vi "Servo_serial_mac_1readwrite.vi"() -> ()   [LabVIEW 2017]
uses:
  <vilib>/Instr/_visa.llb/VISA Configure Serial Port (Instr).vi
panel:
  in  "Pulse Width Input (600-2400)":dbl
  out "Servo Digital Signal":cluster{i32, dbl, dbl[]}(graph)
  out "Position Input":cluster{i32, dbl, dbl[]}(graph)
  out "Digitial Signal":dbl
  in  "Delay":dbl
  in  "Buad Rate":i32(ring) items=["2400"=2400, "4800"=4800, "9600"=9600, "14400"=14400, "19200"=19200, "28800"=28800, "38400"=38400, "57600"=57600, "115200"=115200]
  out "Bytes at port":cluster{i32, dbl, dbl[]}(graph)
  out "Read buffer":string
  in  "Stop":bool
  out "Sent to Arduino":string
  in  "COM Port":refnum<visa-resource-name>
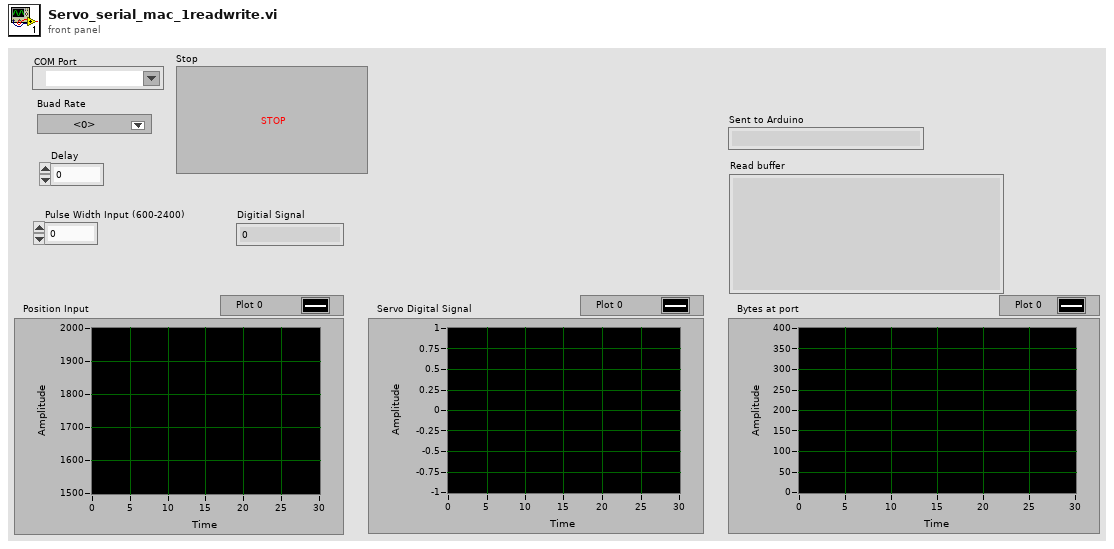
[diagram p1: front panel]
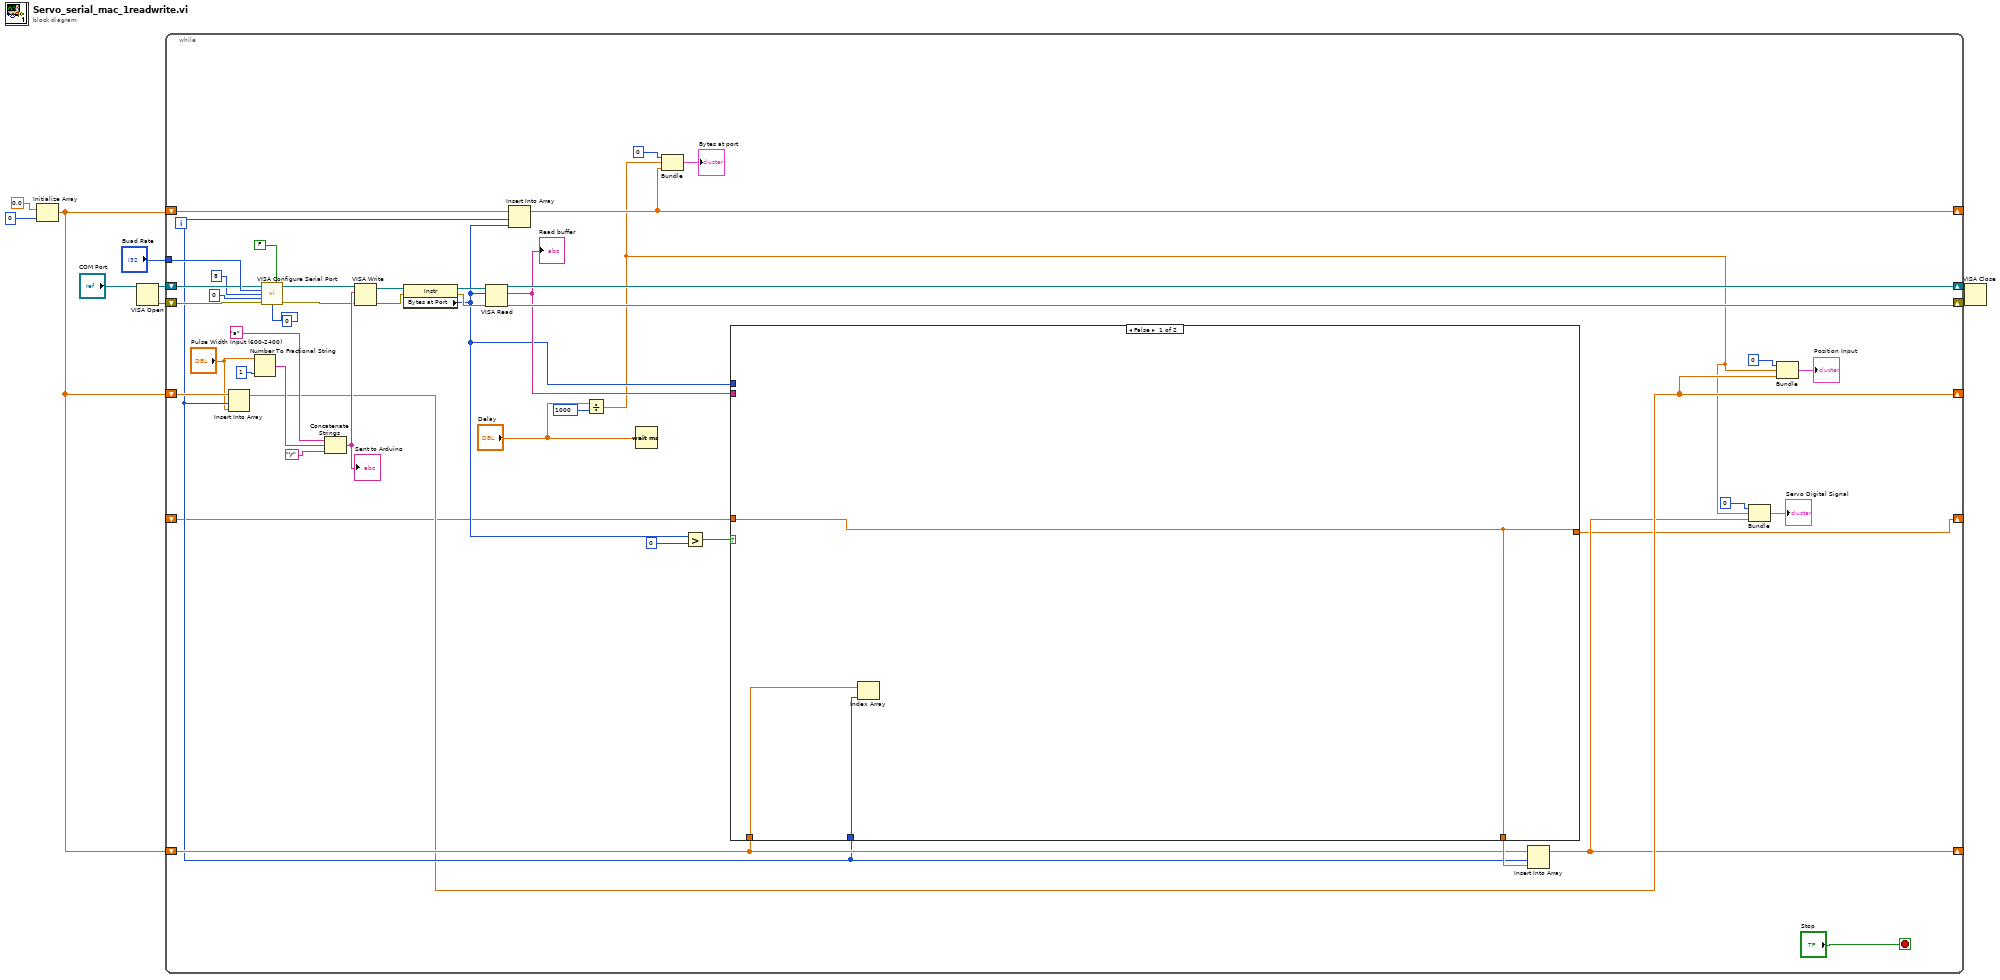
[diagram p0: block diagram]
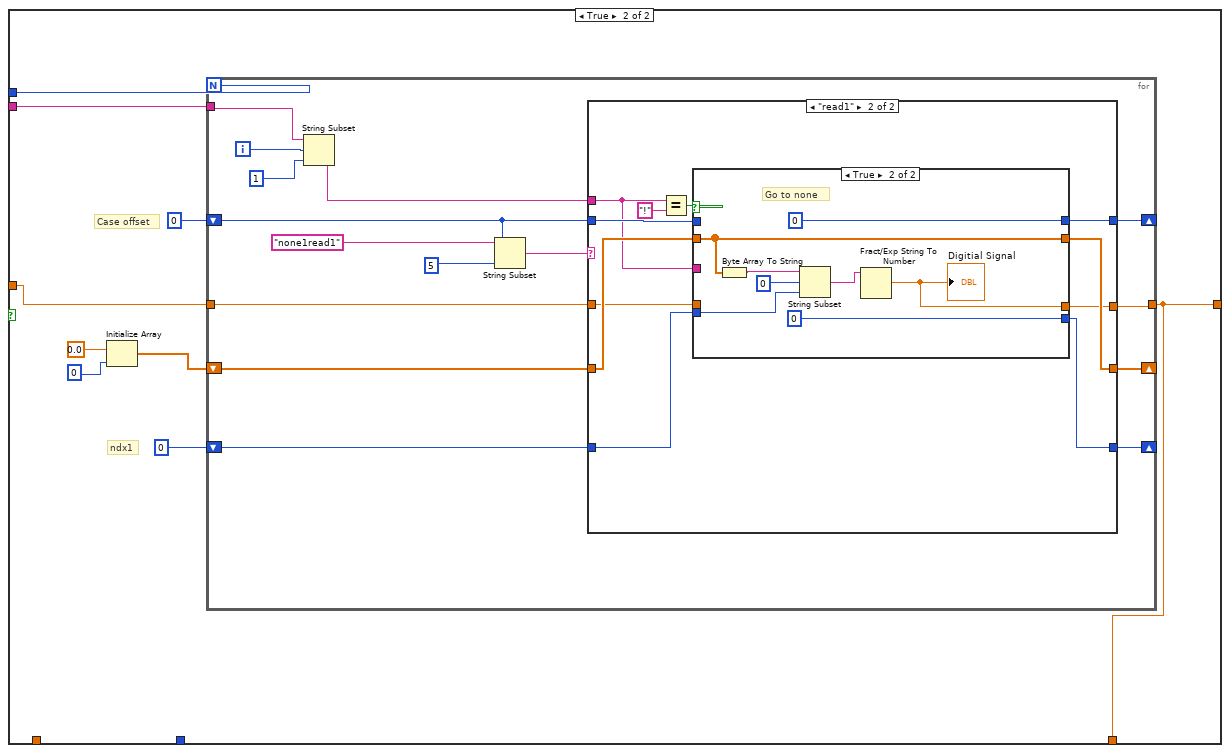
[diagram p2: hidden frame]
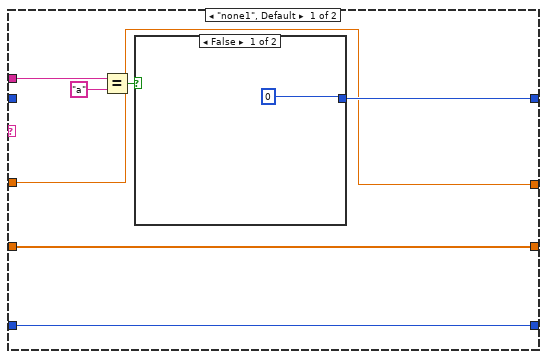
[diagram p3: hidden frame]
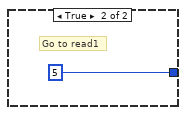
[diagram p4: hidden frame]
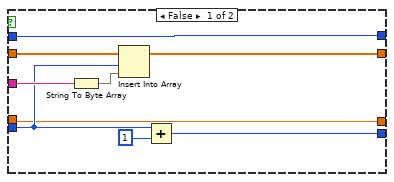
[diagram p5: hidden frame]
diagram:
  n1 = Initialize Array(0.0 ("element"), 0 ("dimension size")) -> (w1:dbl[])
  n2 = VISA Open(VISA resource name="COM Port") -> (VISA resource name=w8:refnum<visa-resource-name>, error out=w7:errorcluster)  [unwired: 4 in]
  n3 = while {
    tunnel: "Buad Rate" -> [w54]
    shift-right: [w50] -> w6
    shift-left: w8 -> [w53]
    shift-right: [w51] -> w5
    shift-left: w7 -> [w52]
    shift-right: [w48] -> _
    shift-left: w1 -> [w49]
    shift-right: [w19] -> _
    shift-left: w1 -> [w28]
    shift-right: [w18] -> _
    shift-left: w1 -> [w24]
    shift-right: [w14] -> _
    shift-left: _ -> [w15]
    i -> [w23]
    stop <- "Stop" stop-if-true
    n4 = Insert Into Array(array=w28, index=w23, new element="Pulse Width Input (600-2400)") -> (w19:dbl[])
    n5 = Number To Fractional String(number="Pulse Width Input (600-2400)", precision (6)=1) -> (F-format string=w44:string)  [unwired: 2 in]
    n6 = call-poly "VISA Configure Serial Port"("VISA resource name"=w53, "Enable Termination\nChar (T)"=FALSE ("Enable Termination\nChar (T)"), "baud rate (9600)"=w54, "data bits (8)"=8, "parity (0:none)"=0, "error in (no error)"=w52, "flow control (0:none)"=0) -> ("VISA resource name out"=w42:refnum<visa-resource-name>, "error out"=w45:errorcluster)  [unwired: 7 in]
    n7 = Concatenate Strings("a", w44, "\r") -> (w46:string)
    "Sent to Arduino" <- w46
    n8 = VISA Write(VISA resource name=w42, write buffer=w46, error in (no error)=w45) -> (VISA resource name out=w38:refnum<visa-resource-name>, error out=w41:errorcluster)  [unwired: 1 out]
    n9 = property class="Instr"(reference=w38, error in=w41) -> (reference out=w39:refnum<visa-resource-name>, error out=w40:errorcluster, "Bytes at Port"=w32:u32)
    n10 = VISA Read(VISA resource name=w39, byte count=w32, error in (no error)=w40) -> (VISA resource name out=w50:refnum<visa-resource-name>, read buffer=w34:string, error out=w51:errorcluster)  [unwired: 1 out]
    "Read buffer" <- w34
    n11 = Insert Into Array(array=w49, index=w23, new element=w32) -> (w48:dbl[])
    n12 = Divide(x="Delay", y=1000) -> (x/y=w17:dbl)
    n13 = Wait (ms)(milliseconds to wait="Delay") -> ()  [unwired: 1 out]
    n14 = Bundle(0, w17, w48) -> (→"Bytes at port":cluster{i32, dbl, dbl[]})  [unwired: 1 in]
    n15 = Greater?(x=w32, y=0) -> (0:w31:bool)
    n16 = case shown="False" w31 {
      tunnel: w32 -> [_ w60]
      tunnel: w34 -> [_ w66]
      tunnel: [w55 w58] -> w25
      tunnel: w23 -> [w56 _]
      tunnel: w24 -> [w57 _]
      tunnel: w15 -> [w55 w59]
      tunnel: [w55 w58] -> w14
      frame False {
        n17 = Index Array(array=w57, index=w56) -> ()  [unwired: 1 out]
      }
      frame True {
        # "ndx1"
        # "Case offset"
        n18 = Initialize Array(0.0 ("element"), 0 ("dimension size")) -> (w61:dbl[])
        n19 = for {
          N: w60 -> [_]
          tunnel: w66 -> [w80]
          shift-right: [w76] -> _
          shift-left: 0 -> [w70]
          shift-right: [w75] -> _
          shift-left: 0 -> [w74]
          shift-right: [w72] -> _
          shift-left: w61 -> [w73]
          tunnel: w59 -> [w67]
          tunnel: [w68] -> w58
          i -> [w69]
          n20 = String Subset(string=w80, offset (0)=w69, length (rest)=1 ("length (rest)")) -> (substring=w77:string)
          n21 = String Subset(string="none1read1", offset (0)=w70, length (rest)=5 ("length (rest)")) -> (substring=w71:string)
          n22 = case shown="\"read1\"" w71 {
            tunnel: w77 -> [w88 w91]
            tunnel: [w85 w98] -> w76
            tunnel: [w84 w94] -> w75
            tunnel: w74 -> [w84 w95]
            tunnel: w73 -> [w82 w96]
            tunnel: [w82 w99] -> w72
            tunnel: w70 -> [_ w97]
            tunnel: [w83 w93] -> w68
            tunnel: w67 -> [w83 w92]
            frame "none1", Default {
              n23 = Equal?(x=w88, y="a") -> (x = y?=w86:bool)
              n24 = case shown="False" w86 {
                tunnel: [0 5] -> w85
                frame False {
                }
                frame True {
                  # "Go to read1"
                }
              }
            }
            frame "read1" {
              n25 = Equal?(x=w91, y="!") -> (x = y?=w100:bool)
              n26 = case shown="True" w100 {
                tunnel: [w110 0] -> w94
                tunnel: w96 -> [w104 w114]
                tunnel: [w108 w114] -> w99
                tunnel: w91 -> [w107 _]
                tunnel: [w105 0] -> w98
                tunnel: w97 -> [w105 _]
                tunnel: w95 -> [w103 w113]
                tunnel: [w102 w111] -> w93
                tunnel: w92 -> [w102 _]
                frame False {
                  n27 = String To Byte Array(string=w107) -> (unsigned byte array=w106:u8[])
                  n28 = Insert Into Array(array=w104, index=w103, new element=w106) -> (w108:dbl[])
                  n29 = Add(x=w103, y=1) -> (x+y=w110:i32)
                }
                frame True {
                  # "Go to none"
                  n30 = Byte Array To String(unsigned byte array=w114) -> (string=w115:string)
                  n31 = String Subset(string=w115, offset (0)=0, length (rest)=w113) -> (substring=w112:string)
                  n32 = Fract/Exp String To Number(string=w112) -> (number=w111:dbl)  [unwired: 3 in, 1 out]
                  "Digitial Signal" <- w111
                }
              }
            }
          }
        }
      }
    }
    n33 = Insert Into Array(array=w24, index=w23, new element=w25) -> (w18:dbl[])
    n34 = Bundle(0, w17, w18) -> (→"Servo Digital Signal":cluster{i32, dbl, dbl[]})  [unwired: 1 in]
    n35 = Bundle(0, w17, w19) -> (→"Position Input":cluster{i32, dbl, dbl[]})  [unwired: 1 in]
  }
  n36 = VISA Close(VISA resource name=w6, error in (no error)=w5) -> ()  [unwired: 1 out]
